vi "printer list com.vi"() -> ()   [LabVIEW 2018]
uses:
  <vilib>/Instr/_visa.llb/VISA Configure Serial Port (Instr).vi
  <vilib>/Utility/file.llb/Read Delimited Spreadsheet (string).vi
panel:
  out "连接的字符串":string
  in  "停止":bool
  in  "发送":bool
  in  "VISA resource name":refnum<visa-resource-name> caption="VISA资源名称"
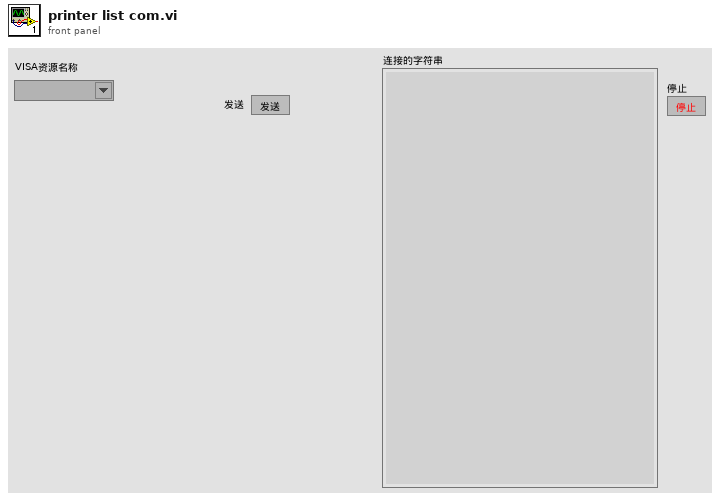
[diagram p1: front panel]
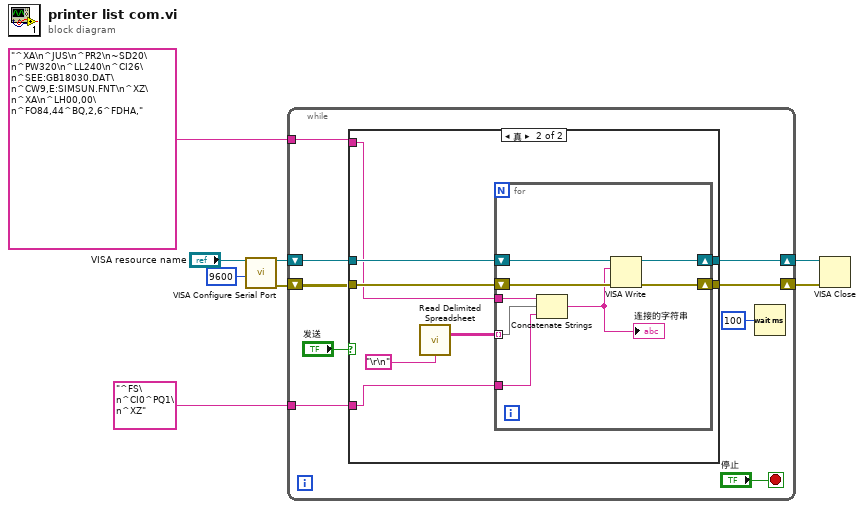
[diagram p0: block diagram]
diagram:
  n1 = call-poly "VISA Configure Serial Port"("VISA resource name"="VISA resource name", "baud rate (9600)"=u32 9600) -> ("VISA resource name out"=w7:refnum<visa-resource-name>, "error out"=w5:errorcluster)  [unwired: 12 in]
  n2 = while {
    shift-right: [w16] -> w6
    shift-left: w7 -> [w17]
    shift-right: [w14] -> w4
    shift-left: w5 -> [w15]
    tunnel: "^XA\n^JUS\n^PR2\n~SD20\n^PW320\n^LL240\n^CI26\n^SEE:GB18030.DAT\n^CW9,E:SIMSUN.FNT\n^XZ\n^XA\n^LH00,00\n^FO84,44^BQ,2,6^FDHA," -> [w10]
    tunnel: "^FS\n^CI0^PQ1\n^XZ" -> [w9]
    stop <- "停止" stop-if-true
    n3 = case shown="真" "发送" {
      tunnel: w17 -> [w19 w27]
      tunnel: [w19 w26] -> w16
      tunnel: w15 -> [w18 w25]
      tunnel: [w18 w24] -> w14
      tunnel: w10 -> [_ w22]
      tunnel: w9 -> [_ w21]
      frame False {
      }
      frame True {
        n4 = call-poly <vilib>:"Read Delimited Spreadsheet.vi"("delimiter (\\t)"="\r\n") -> ("all rows"=w20:string[][])  [unwired: 9 in, 5 out]
        n5 = for {
          tunnel: w22 -> [w31]
          shift-right: [w34] -> w26
          shift-left: w27 -> [w35]
          shift-right: [w32] -> w24
          shift-left: w25 -> [w33]
          tunnel: w20 -> [w29] mode=indexing
          tunnel: w21 -> [w28]
          n6 = Concatenate Strings(w31, w29, w28) -> (w30:string)
          "连接的字符串" <- w30
          n7 = VISA Write(VISA resource name=w35, write buffer=w30, error in (no error)=w33) -> (VISA resource name out=w34:refnum<visa-resource-name>, error out=w32:errorcluster)  [unwired: 1 out]
        }
      }
    }
    n8 = Wait (ms)(milliseconds to wait=u32 100 ("等待时间（毫秒）")) -> ()  [unwired: 1 out]
  }
  n9 = VISA Close(VISA resource name=w6, error in (no error)=w4) -> ()  [unwired: 1 out]
